vi "SEM HV log.vi"(8 "error in":errorcluster, 10 "SEM HV DataLog Files Directory":path=path "D:/3D FIB-SEM Files/SEM HV DataLog", 11 "ActiveX Container":refnum<k7>(container)) -> (0 "error out":errorcluster, 2 "SEM HV Data Output":T1 {"Sys Vac (Torr)" format="%.2e"; "Gun Vac (Torr)" format="%.2e"; "Supp Monitor (V)" format="%.1f"; "Liner Actual (V)" format="%.1f"; "Fil I Actual (A)" format="%.3f"; "Ext Actual (V)" format="%.1f"; "Supp Actual (V)" format="%.1f"; "EHT Actual (V)" format="%.1f"; "EHT Target (V)" format="%.1f"; "Liner Target (V)" format="%.1f"; "Fil I Target (A)" format="%.3f"; "Fil Age (hr)" format="%.2f"; "Ext I Actual (uA)" format="%.1f"; "Ext Target (V)" format="%.1f"}, 3 "reference out":refnum<k7>)   [LabVIEW 2018]
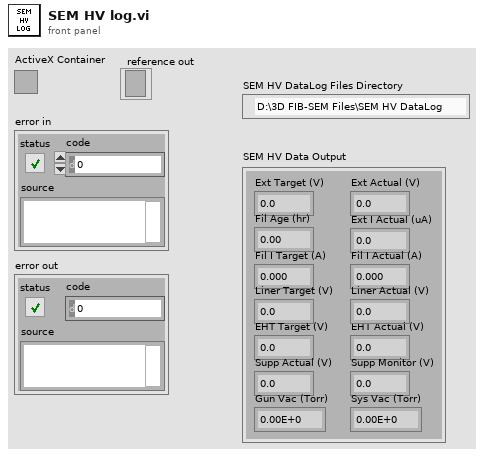
[diagram p1: front panel]
types:
  T1 = cluster{"Ext Target (V)":sgl, "Ext Actual (V)":sgl, "Fil Age (hr)":sgl, "Ext I Actual (uA)":sgl, "Fil I Target (A)":sgl, "Fil I Actual (A)":sgl, "Liner Target (V)":sgl, "Liner Actual (V)":sgl, "EHT Target (V)":sgl, "EHT Actual (V)":sgl, "Supp Actual (V)":sgl, "Supp Monitor (V)":sgl, "Gun Vac (Torr)":sgl, "Sys Vac (Torr)":sgl}
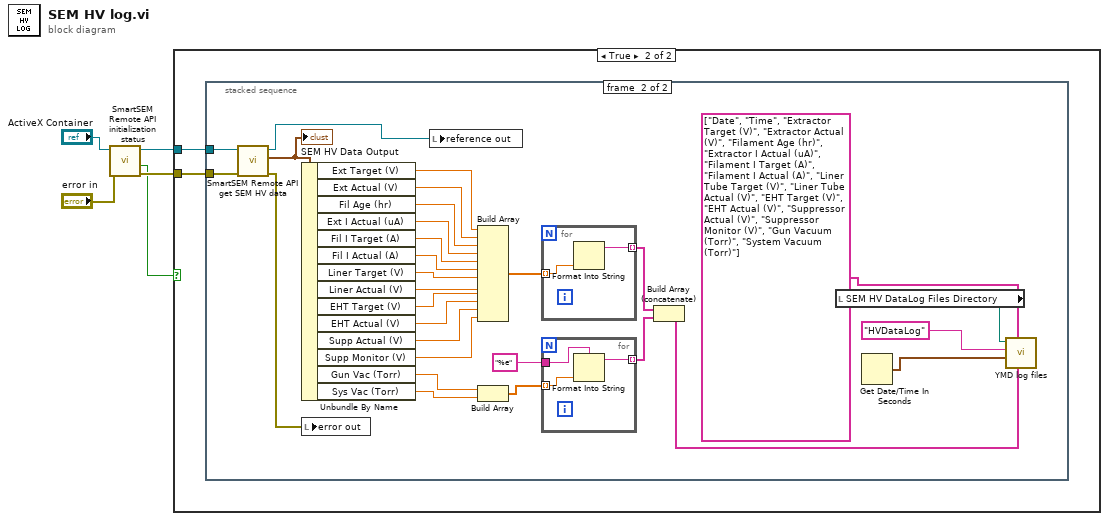
[diagram p0: block diagram]
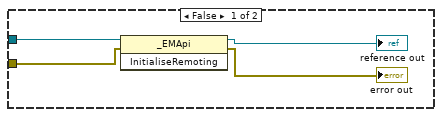
[diagram p2: hidden frame]
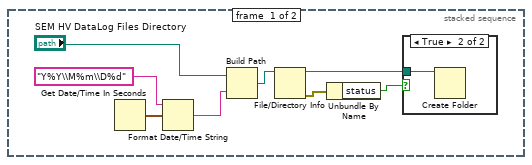
[diagram p3: hidden frame]
diagram:
  n1 = call "SmartSEM Remote API initialization status.vi"("error in"="error in", "ActiveX Container"="ActiveX Container") -> ("error out"=w4:errorcluster, "API initialized"=w3:bool, "reference out"=w5:refnum<k7>)  [unwired: 7 in]
  n2 = case shown="True" w3 {
    tunnel: w5 -> [w9 w11]
    tunnel: w4 -> [w7 w10]
    frame False {
      n3 = invoke class="_EMApi" method="InitialiseRemoting"(reference=w9, error in=w7) -> (reference out=→"reference out":refnum<k7>, error out=→"error out":errorcluster)  [unwired: 1 in, 1 out]
    }
    frame True {
      n4 = stacked-sequence {
        tunnel: w11 -> [_ w24]
        tunnel: w10 -> [_ w23]
        frame #0 {
          n5 = Get Date/Time In Seconds() -> (seconds since 1Jan1904=w19:timestamp)
          n6 = Format Date/Time String(time format string (%c)="Y%Y\\M%m\\D%d", seconds (now)=w19) -> (date/time string=w15:string)  [unwired: 1 out]
          n7 = Build Path(base path="SEM HV DataLog Files Directory", name or relative path=w15) -> (appended path=w13:path)
          n8 = File/Directory Info(path=w13) -> (path out=w18:path, error out=w16:errorcluster)  [unwired: 1 in, 5 out]
          n9 = Unbundle By Name(w16) -> ("status"=w17:bool)
          n10 = case shown="True" w17 {
            tunnel: w18 -> [_ w20]
            frame False {
            }
            frame True {
              n11 = Create Folder(path (use dialog)=w20) -> ()  [unwired: 1 in, 4 out]
            }
          }
        }
        frame #1 {
          n12 = call "SmartSEM Remote API get SEM HV data.vi"("error in"=w23, "ActiveX Container"=w24) -> ("error out"=w21:errorcluster, "SEM HV Data Output"=w26:T1, "reference out"=w22:refnum<k7>)  [unwired: 7 in]
          "SEM HV Data Output" <- w26
          n13 = Unbundle By Name(w26) -> ("Ext Target (V)"=w31:sgl, "Ext Actual (V)"=w32:sgl, "Fil Age (hr)"=w33:sgl, "Ext I Actual (uA)"=w34:sgl, "Fil I Target (A)"=w35:sgl, "Fil I Actual (A)"=w36:sgl, "Liner Target (V)"=w43:sgl, "Liner Actual (V)"=w42:sgl, "EHT Target (V)"=w37:sgl, "EHT Actual (V)"=w38:sgl, "Supp Actual (V)"=w39:sgl, "Supp Monitor (V)"=w40:sgl, "Gun Vac (Torr)"=w25:sgl, "Sys Vac (Torr)"=w44:sgl)
          n14 = local write "error out"(w21) -> ()
          n15 = local write "reference out"(w22) -> ()
          n16 = Build Array(w31, w32, w33, w34, w35, w36, w43, w42, w37, w38, w39, w40) -> (w41:sgl[])
          n17 = Build Array(w25, w44) -> (w45:sgl[])
          n18 = for {
            tunnel: w41 -> [w54] mode=indexing
            tunnel: [w53] -> w47 mode=indexing
            n19 = Format Into String(w54) -> (resulting string=w53:string)  [unwired: 3 in, 1 out]
          }
          n20 = for {
            tunnel: w45 -> [w52] mode=indexing
            tunnel: [w51] -> w48 mode=indexing
            tunnel: "%e" ("format string") -> [w50]
            n21 = Format Into String(format string=w50, w52) -> (resulting string=w51:string)  [unwired: 2 in, 1 out]
          }
          n22 = Build Array (concatenate)(w47, w48) -> (w49:string[])
          n23 = local read "SEM HV DataLog Files Directory"() -> (w28:path)
          n24 = Get Date/Time In Seconds() -> (seconds since 1Jan1904=w29:timestamp)
          n25 = call "YMD log files.vi"("Input text array"=w49, "Input header array"=string[] ["Date", "Time", "Extractor Target (V)", "Extractor Actual (V)", "Filament Age (hr)", "Extractor I Actual (uA)", "Filament I Target (A)", "Filament I Actual (A)", "Liner Tube Target (V)", "Liner Tube Actual (V)", "EHT Target (V)", "EHT Actual (V)", "Suppressor Actual (V)", "Suppressor Monitor (V)", "Gun Vacuum (Torr)", "System Vacuum (Torr)"], "current time"=w29, "Log file name"="HVDataLog" ("string"), "Log file path"=w28) -> ()  [unwired: 7 in]
        }
      }
    }
  }
